vi "Build.vi"(0 "NIPKG_LV In":refnum<class "NIPKG_LV.lvclass">) -> (4 "NIPKG_LV Out":refnum<class "NIPKG_LV.lvclass">)   [LabVIEW 2017, in "CL_G3_VIComponentBuilder.lvlib" / "NIPKG_LV.lvclass"]
doc: "Adds the newly created NI Package to the build machine feed. Creates the buld machine folder path if it does not already exist."
uses:
  NIPKG_LV.lvclass
  C:/builds/Component BuilderBT/SrcDist/Exports/Exports/Export.lvclass
  Exports/Export.lvclass/Export.ctl
  NIPKG_LV.lvclass/NIPKG_LV.ctl
  Exports/Accessors/Write Export Operation Errors.vi
  Exports/Accessors/Read Export Operation Errors.vi
  Accessors/Read Build Machine Feed Folderpath.vi
  Exports/Accessors/Read Built Export's Full Path.vi
  NI Build Specification_LV/NI Build Specification_LV.lvclass
  <userlib>/_Cirrus Logic/NI Package Manager API/Source/TCS_NIPKG_API.lvlib
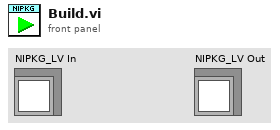
[diagram p1: front panel]
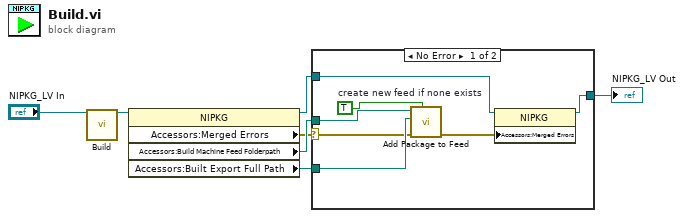
[diagram p0: block diagram]
diagram:
  n1 = call-parent "Build.vi"("NI Build Specification_LV In"="NIPKG_LV In") -> ("NI Build Specification_LV Out"=w3:refnum<class "NIPKG_LV.lvclass">)  [unwired: 14 in]
  n2 = property class="NIPKG"(reference=w3) -> (reference out=w5:refnum<class "NIPKG_LV.lvclass">, "Accessors:Merged Errors"=w1:errorcluster, "Accessors:Build Machine Feed Folderpath"=w6:path, "Accessors:Built Export Full Path"=w4:path)  [unwired: 1 in, 1 out]
  n3 = case shown="No Error" w1 {
    selector: w1 -> [w8 _]
    tunnel: w6 -> [w14 _]
    tunnel: w5 -> [w13 w15]
    tunnel: w4 -> [w12 _]
    tunnel: [w10 w15] -> w2
    frame No Error {
      w11 = TRUE  # create new feed if none exists
      n4 = call <userlib>:"Add Package to Feed.vi"("create new feed if none exists (F)"=w11, "error in"=w8, "package source filepath"=w12, "feed folderpath"=w14) -> ("error out"=w9:errorcluster)  [unwired: 7 in]
      n5 = property class="NIPKG"(reference=w13, "Accessors:Merged Errors"=w9) -> (reference out=w10:refnum<class "NIPKG_LV.lvclass">)  [unwired: 1 in, 1 out]
    }
    frame Error {
    }
  }
  "NIPKG_LV Out" <- w2
